vi "Periodic Tasks.vi"(8 "error in":errorcluster) -> ()   [LabVIEW 2016]
doc: "This VI runs in parallel to other tasks. It can contain as many user-defined periodic loops as you need. These can carry out PID or other sorts of timed response."
uses:
  <vilib>/Rock Robotics/WPI/Solenoid/WPI_SolenoidValue.ctl
  <vilib>/Rock Robotics/WPI/Utilities/WPI_GetSetVariantRefNum.vi
  Robot Global Data.vi
  <vilib>/addons/control/pid/pid.llb/PID (DBL).vi
  <vilib>/Rock Robotics/WPI/RobotDrive/WPI_RobotDriveMecanumDrive_Cartesian.vi
  <vilib>/Rock Robotics/WPI/Solenoid/WPI_SolenoidSetEnum.vi
  <vilib>/Rock Robotics/Network Tables/NT Read Number.vi
  <vilib>/Rock Robotics/Network Tables/NT Write Boolean.vi
  navX Library v2/navX Library v2.lvlib
  <vilib>/Analysis/NI_AALBase.lvlib
  <vilib>/addons/control/pid/NI_PID_pid.lvlib
panel:
  in  "gearDepthresh left":dbl=1.92 format="%#_13g"
  out "target angle":dbl
  in  "cam FOV":dbl=34.0 format="%#_13g"
  out "panic":bool
  out "YavSaved":dbl=162.56
  in  "PID Strafe Straight":T1={"proportional gain (Kc)"=0.05, "integral time (Ti, min)"=0.007, "derivative time (Td, min)"=0.001} {"derivative time (Td, min)" format="%.3f"; "integral time (Ti, min)" format="%.3f"; "proportional gain (Kc)" format="%.3f"}
  in  "min thresh 2":dbl=5e-05 format="%#_13g"
  in  "add if slow 2":dbl=0.005 format="%#_13g"
  in  "add if fast 2":dbl format="%#_13g"
  in  "min thresh":dbl=5e-05 format="%#_13g"
  in  "add if slow":dbl=0.005 format="%#_13g"
  in  "add if fast":dbl format="%#_13g"
  in  "aim thresh fast to mid":dbl=90.0
  out "turnSpeedSlow working":dbl=0.18
  out "turnSpeedStartSlow working":dbl=0.17
  in  "turnSpeedMedium":dbl=0.2 format="%#_13g"
  in  "turnSpeedHard":dbl=0.25 format="%#_13g"
  in  "cameraTarget":dbl=-0.195 format="%#_13g"
  in  "aim thresh start as slow":dbl=15.0 format="%#_13g"
  in  "turnSpeedSlow":dbl=0.19 format="%#_13g"
  in  "turnSpeedStartSlow":dbl=0.19
  out "aimState":i32
  out "leftOrRight":dbl=1.0
  in  "aim thresh mid to slow":dbl=30.0
  out "aimBot":dbl
  in  "hopperSpeedClose":dbl=0.5 step=0.05
  in  "Kd 2":dbl
  in  "Ki 2":dbl
  in  "Kp 2":dbl
  in  "armPanic Thresh":dbl=1.0
  in  "gearDepthresh right":dbl=1.92 format="%#_13g"
  out "std dev":dbl=3.505907882345
  out "mean":dbl=4.613466334164588
  in  "gearSensthresh":dbl=1.15 format="%#_13g"
  out "Input Voltage":dbl=10.350000000000001
  out "voltage (V)":dbl=10.15
  in  "SHIMMYTIME2":i32=10
  in  "SHIMMYTIME1":i32=10
  out "Waveform Graph":dbl[](graph)=[0.0, 0.0, 0.0, 0.0, 0.0, 0.0, 0.0, 0.0, 0.0, 0.0, 0.0, 0.0, 0.0, 0.0, 0.0, 0.0, 0.0, 0.0, 0.0, 0.0, 0.0, 0.0, 0.0, 0.0, 0.0, 0.0, 0.0, 0.0, 0.0, 0.0, 0.0, 0.0, 0.0, 0.0, 0.0, 0.0, 0.0, 0.0, 0.0, 0.0, 0.0, 0.0, 0.0, 0.0, 0.0, 0.0, 0.0, 0.0, 0.0, 0.0, 0.0, 0.0, 0.0, 0.0, 0.0, 0.0, 0.0, 0.0, 0.0, 0.0, 0.0, 0.0, 0.0, 0.0, 0.0, 0.0, 0.0, 0.0, 0.0, 0.0, 0.0, 0.0, 0.0, 0.0, 0.0, 0.0, 0.0, 0.0, 0.0, 0.0, 0.0, 0.0, 0.0, 0.0, 0.0, 0.0, 0.0, 0.0, 0.0, 0.0, 0.0, 0.0, 0.0, 0.0, 0.0, 0.0, 0.0, 0.0, 0.0, 0.0, 0.0, 0.0, 0.0, 0.0, 0.0, 0.0, 0.0, 0.0, 0.0, 0.0, 0.0, 0.0, 0.0, 0.0, 0.0, 0.0, 0.0, 0.0, 0.0, 0.0, 0.0, 0.0, 0.0, 0.0, 0.0, 0.0, 0.0, 0.0, 0.0, 0.0, 0.0, 0.0, 0.0, 0.0, 0.0, 0.0, 0.0, 0.0, 0.0, 0.0, 0.0, 0.0, 0.0, 0.0, 5.625, 5.875, 6.125, 6.0, 6.0, 6.0, 7.0, 8.0, 7.5, 7.0, 6.75, 6.5, 6.625, 6.25, 9.625, 10.25, 6.875, 6.625, 6.75, 7.125, 6.875, 6.875, 6.875, 7.0, 6.625, 7.125, 6.625, 6.375, 6.875, 7.5, 7.125, 7.875, 8.75, 8.25, 6.75, 7.375, 7.125, 7.375, 7.125, 7.125, 6.625, 6.5, 7.0, 7.0, 7.0, 6.75, 7.125, 7.625, 7.0, 7.75, 7.0, 7.125, 6.625, 7.25, 6.625, 6.75, 6.75, 6.75, 6.75, 7.0, 6.5, 6.75, 7.625, 7.25, 7.25, 7.25, 6.5, 7.0, 6.875, 7.125, 7.0, 7.25, 7.375, 6.875, 6.625, 6.625, 7.25, 6.5, 7.0, 6.75, 6.375, 6.75, 6.75, 6.875, 6.75, 6.75, 6.875, 6.25, 7.0, 6.375, 6.375, 6.875, 7.0, 6.5, 7.875, 8.5, 6.75, 6.625, 7.0, 7.0, 6.875, 7.0, 6.875, 8.125, 7.375, 6.75, 6.5, 6.375, 6.375, 6.875, 6.75, 7.0, 7.125, 7.125, 6.875, 7.0, 7.125, 7.875, 7.875, 8.75, 8.25, 7.0, 7.625, 7.0, 7.25, 7.125, 7.25, 7.0, 6.875, 7.0, 6.875, 7.25, 7.75, 7.625, 7.25, 7.125, 8.0, 8.75, 7.25, 7.125, 8.125, 10.125, 9.5, 8.75, 7.0, 6.875, 6.75, 6.875, 6.75, 7.25, 7.0, 8.25, 7.875, 7.5, 7.875, 6.75, 6.75, 7.875, 8.0, 8.375, 7.0, 6.75, 8.75, 7.875, 7.5, 7.5, 8.5, 7.0, 6.75, 7.125, 7.5, 7.375, 7.625, 7.25, 7.0, 6.875, 7.0, 7.125, 7.125, 8.25, 7.625, 7.125, 7.375, 7.125, 7.0, 7.875, 6.875, 7.0, 7.25, 7.25, 6.75, 6.875, 7.5, 6.5, 7.0, 6.875, 6.75, 6.875, 7.0, 6.875, 7.0, 7.25, 7.75, 7.875, 6.75, 6.875, 7.375, 7.125, 6.625, 7.625, 7.0, 7.25, 7.125, 7.125, 7.25, 7.25, 7.5, 6.875, 6.75, 7.0, 6.75, 6.125, 7.125, 6.75, 6.75, 6.875, 7.875, 7.125, 7.375, 7.0, 6.625, 6.75, 7.875, 9.25, 10.125, 7.625, 7.125, 6.625, 7.125, 8.625, 8.5, 7.375, 7.0, 7.0, 7.375, 11.5, 6.875, 7.125, 6.875, 6.875, 7.5, 7.5, 7.625, 7.375, 6.875, 7.125, 7.25]
  in  "Kd":dbl
  in  "Ki":dbl
  in  "Kp":dbl
  in  "ARM Retainer open":bool
  in  "SEQ Retainer Open":bool
  in  "Gear Shover":bool
  in  "Ramp-Up":dbl format="%#_13g"
  out "Shooter Speed":dbl
  out "trim close":dbl=1.0009448818897637
  out "trim far":dbl=1.0003149606299213
  out "timeSaved 2":i32=400
  in  "drop gear time":i32=40
  in  "open retainer time":i32=20
  in  "shooter target speed close":dbl=6.5 format="%.2f"
  in  "feed forward close":dbl=0.66 step=0.05
  in  "shooter target speed far":dbl=7.0 format="%.2f"
  out "timeSaved":i32=41241
  in  "shimmyspeed":dbl=0.3
  in  "xshimmy":bool
  in  "intakeSpeed":dbl=0.8
  in  "Slews":cluster{"slewX":dbl, "slewYgo":dbl, "slewZ":dbl}={"slewX"=0.2, "slewYgo"=0.2, "slewZ"=0.15}
  # "DRIVE STUFF"
  # "BALL STUFF"
  # "GEAR STUFF"
  # ".5"
  # "2/16:\nFF far:      0.71\nFF Close: 0.66\nKp Far = 0.025\nTarget speed far = 7"
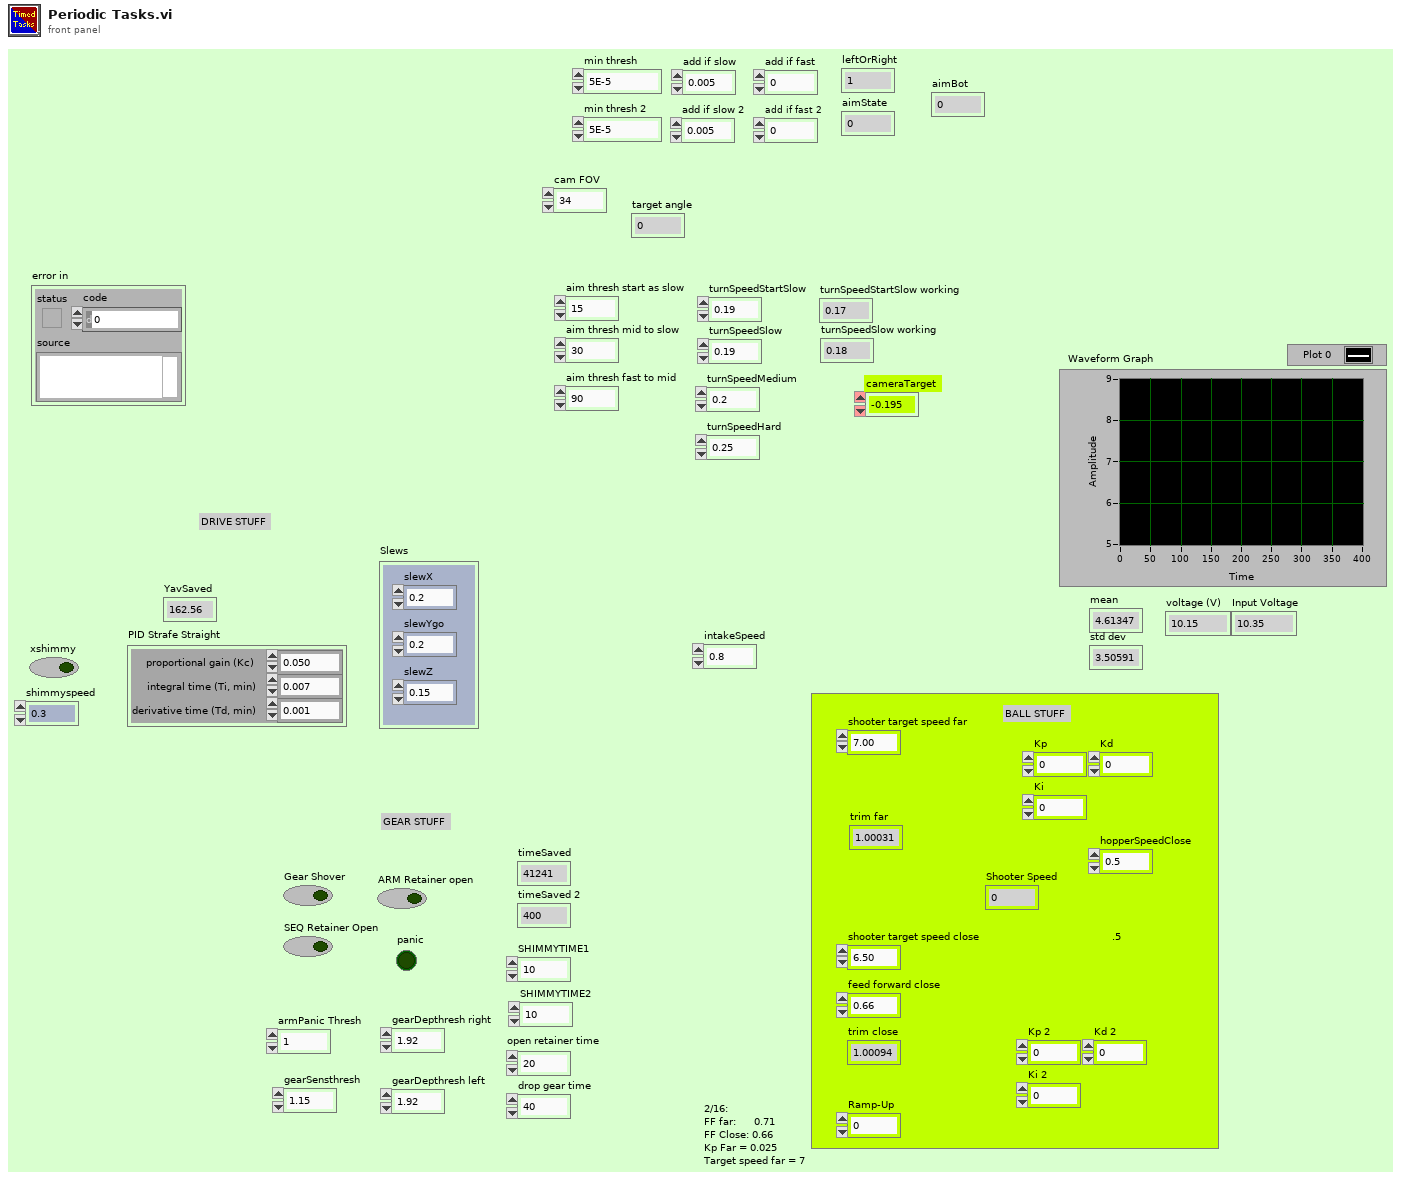
[diagram p1: front panel]
types:
  T1 = cluster{"proportional gain (Kc)":dbl, "integral time (Ti, min)":dbl, "derivative time (Td, min)":dbl}
  T2 = typedef "WPI_SolenoidDevRef.ctl" = cluster{"DevStatus":errorcluster, "Pneumatics Control Module":u8, "Forward Solenoid Channel":T3, "Reverse Solenoid Channel":T3}
  T3 = typedef "WPI_SolenoidChannel.ctl" = enum8{"Solenoid 0", "Solenoid 1", "Solenoid 2", "Solenoid 3", "Solenoid 4", "Solenoid 5", "Solenoid 6", "Solenoid 7", "Invalid"}
  T4 = typedef "navX Library v2.lvlib/Z900_navX_DeviceTypeDef.ctl" = cluster{"Interface":cluster{"Protocol":T5, "Update Rate (4Hz-100Hz)":u8, "navX Open TypeDef":variant}, "Notify Packet":refnum<notifier>, "Loop VI Refnum":refnum<vi>, "Ready to Close Occurrence Refnum":refnum<k4>}
  T5 = typedef "navX Library v2.lvlib/Z900_navX_ProtocolTypeDef.ctl" = enum16{"SERIAL", "I2C", "SPI"}
  T6 = typedef "WPI_EncoderDevRef.ctl" = cluster{"DevStatus":errorcluster, "EncoderIndex":T7, "CounterIndex":T8, "DistancePerCount":dbl, "Decoding Type":T9}
  T7 = typedef "FPGA_EncoderIdx.ctl" = enum8{"Enc 0", "Enc 1", "Enc 2", "Enc 3", "Enc 4", "Enc 5", "Enc 6", "Enc 7", "Invalid"}
  T8 = typedef "FPGA_CounterCtrSystemIndex.ctl" = enum8{"Ctr 0", "Ctr 1", "Ctr 2", "Ctr 3", "Ctr 4", "Ctr 5", "Ctr 6", "Ctr 7", "Invalid"}
  T9 = typedef "WPI_EncoderType.ctl" = enum16{"1x", "2x", "4x"}
  T10 = typedef "WPI_MotorControlDeviceRef.ctl" = cluster{"DeviceStatus":errorcluster, "Type":T11, "PWM":cluster{"PWM Channel":T12, "DeadBand":T13}, "CAN":cluster{"Device Number":u8, "SetOutput VI Ref":variant, "GetOutput VI Ref":variant, "Enable VI Ref":variant, "Disable VI Ref":variant, "Data":variant}, "Invert":bool}
  T11 = typedef "WPI_MotorControlType.ctl" = enum16{"PWM", "CAN"}
  T12 = typedef "FPGA_DIOPWMChannel.ctl" = enum8{"PWM 0", "PWM 1", "PWM 2", "PWM 3", "PWM 4", "PWM 5", "PWM 6", "PWM 7", "PWM 8", "PWM 9", "PWM MXP 0", "PWM MXP 1", "PWM MXP 2", "PWM MXP 3", "PWM MXP 4", "PWM MXP 5", "PWM MXP 6", "PWM MXP 7", "PWM MXP 8", "PWM MXP 9", "Invalid"}
  T13 = typedef "WPI_PWMDeadband.ctl" = cluster{"Name":string, "maxPositivePwm":i32, "minPositivePwm":i32, "centerPwm":i32, "maxNegativePwm":i32, "minNegativePwm":i32, "angularRange":u16}
  T14 = typedef "WPI_CompressorDevRef.ctl" = cluster{"DevStatus":errorcluster, "Pneumatics Control Module":u8}
  T15 = typedef "WPI_RobotDriveDevRef.ctl" = cluster{"DevStatus":errorcluster, "Motors[]":T10[], "Square Inputs":bool, "Max Output":dbl}
  T16 = typedef "WPI_AnalogChannelDevRef.ctl" = cluster{"DevStatus":errorcluster, "Analog Channel":T17}
  T17 = typedef "FPGA_AIChannel.ctl" = enum8{"AI 0", "AI 1", "AI 2", "AI 3", "AI MXP 0", "AI MXP 1", "AI MXP 2", "AI MXP 3", "Invalid"}
  T18 = cluster{"Yaw":dbl, "Roll":dbl, "Pitch":dbl, "Heading":dbl, "Fused Heading":dbl}
  T19 = typedef "WPI_SolenoidValue.ctl" = enum16{"Off", "On", "Forward", "Reverse"}
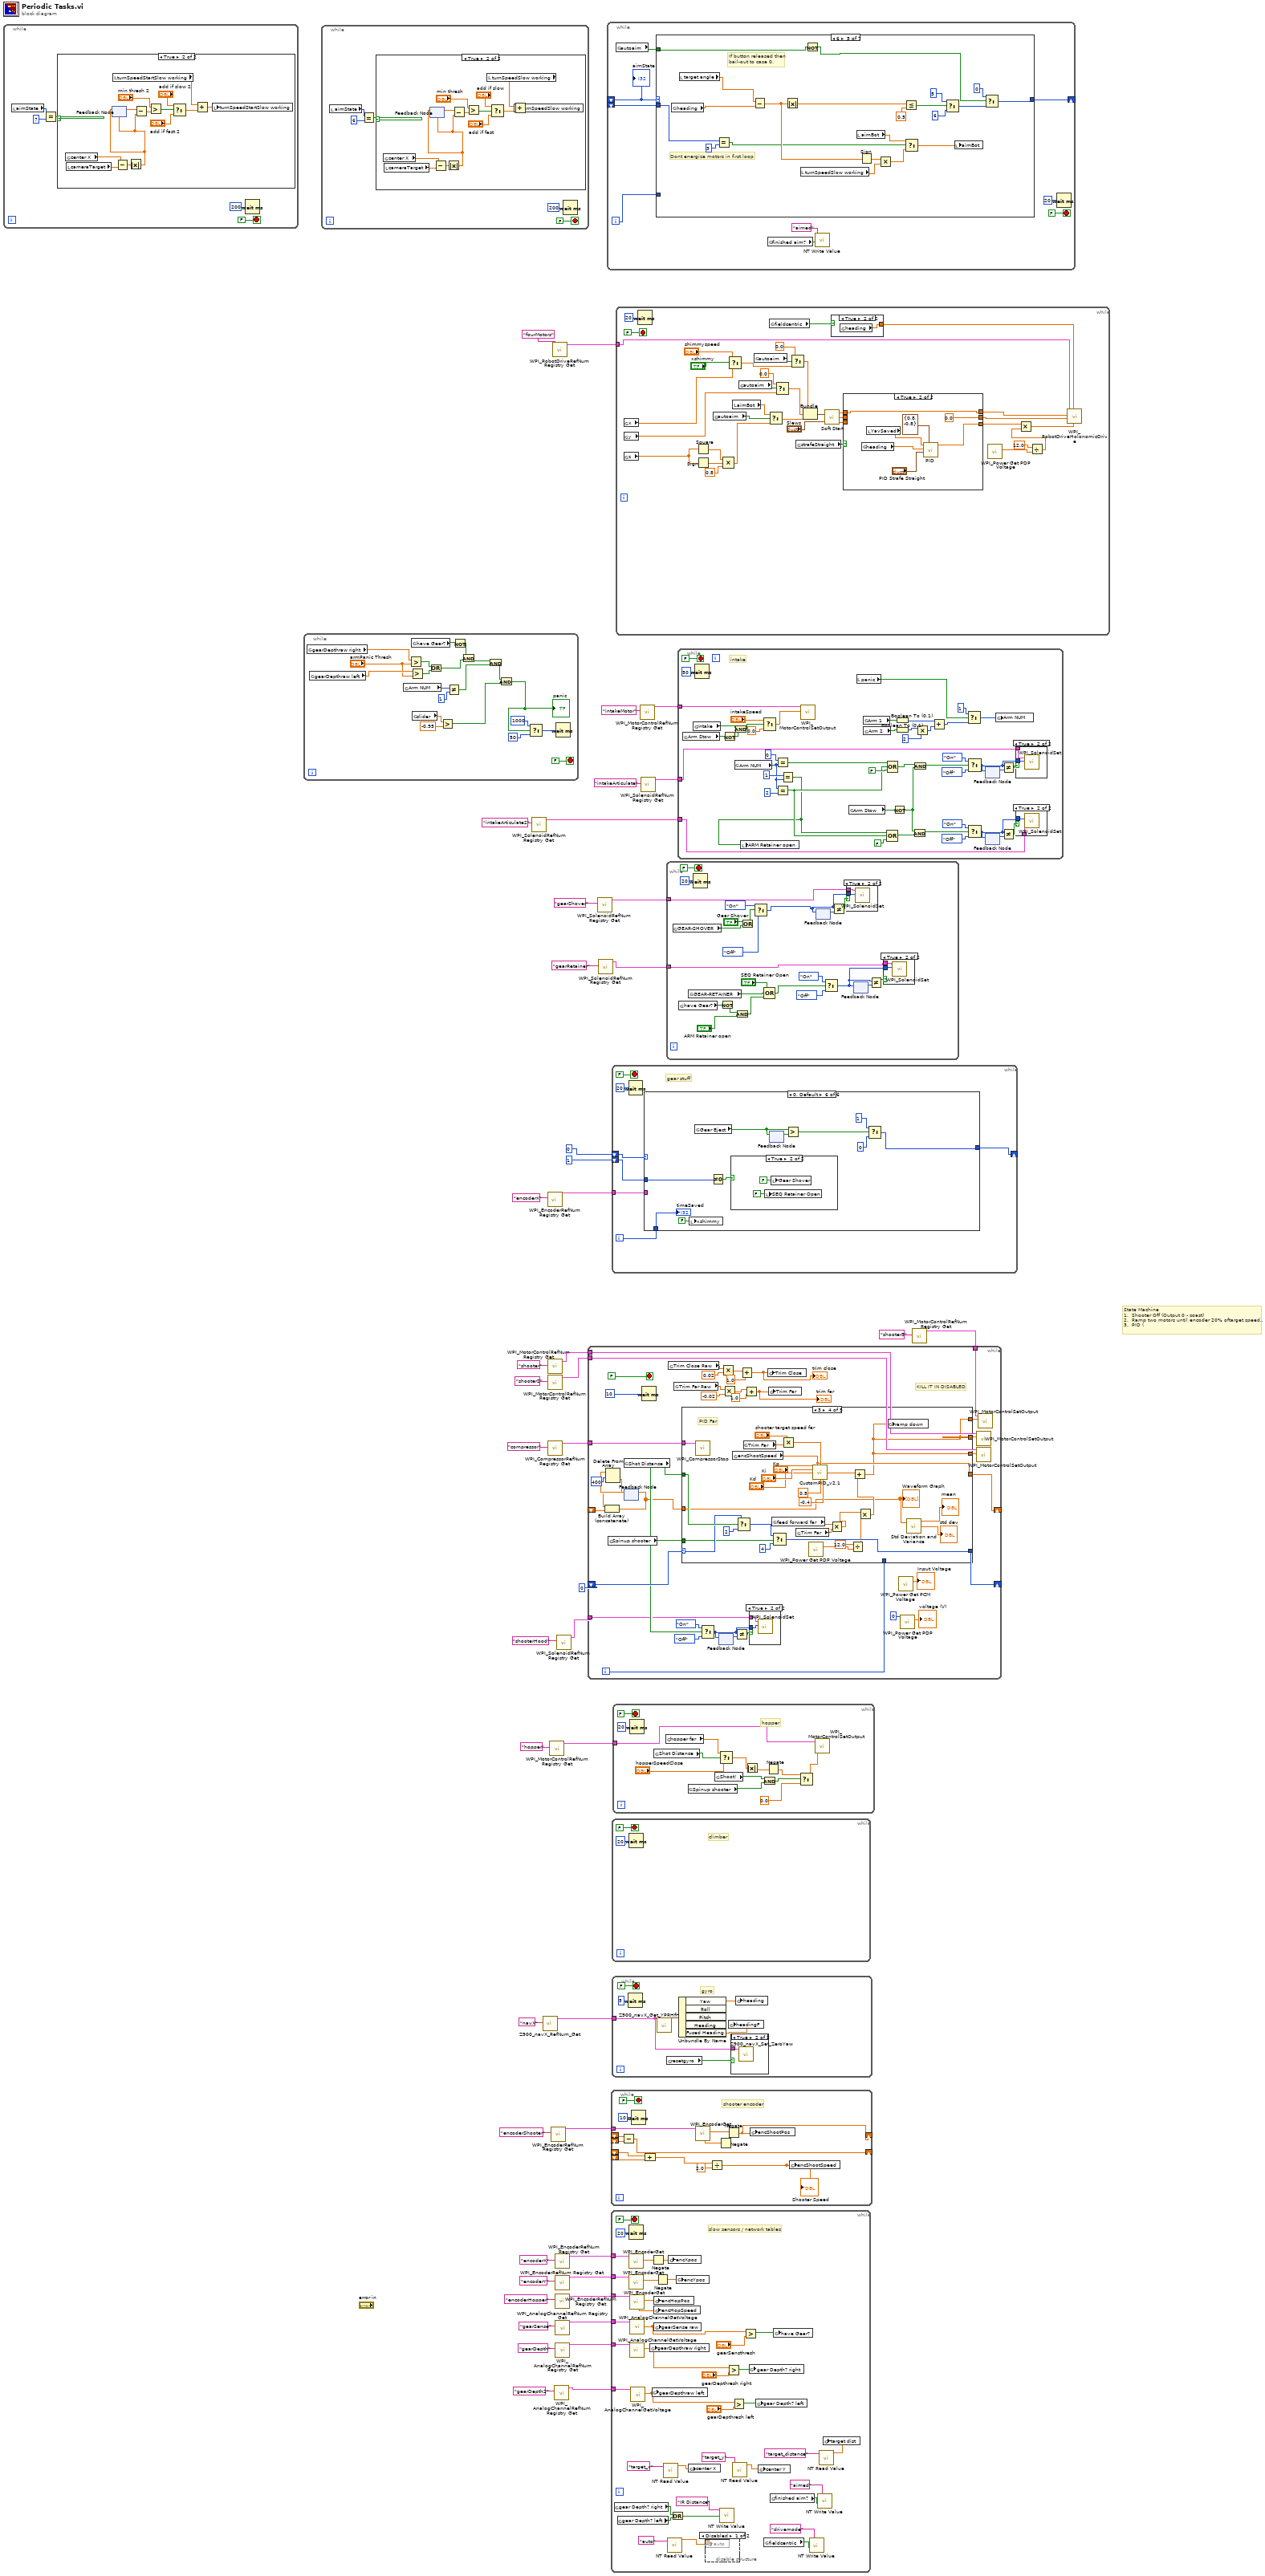
[diagram p0: block diagram]
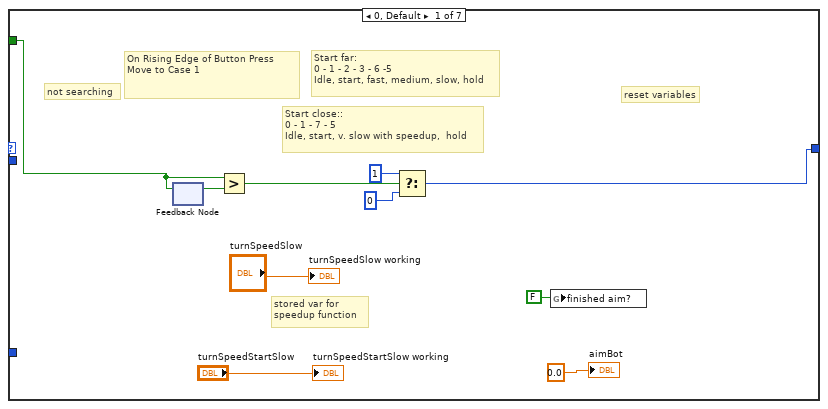
[diagram p4: hidden frame]
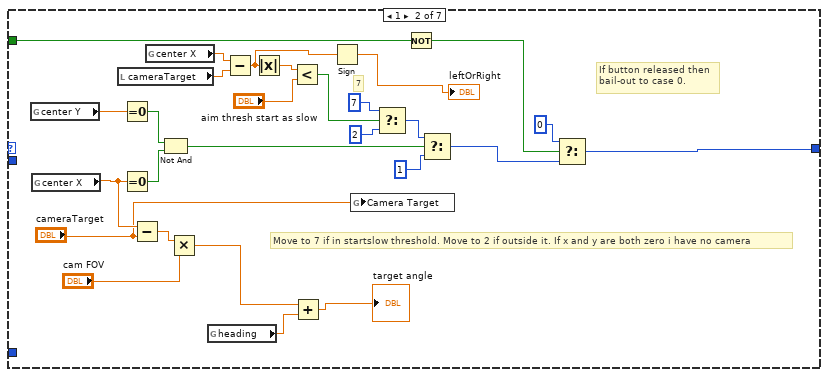
[diagram p5: hidden frame]
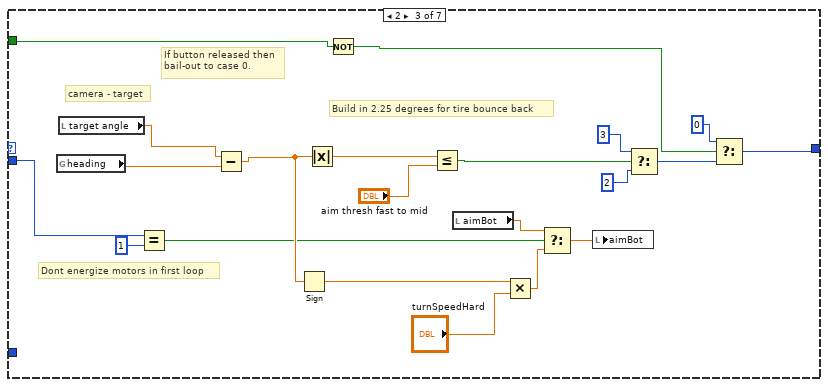
[diagram p6: hidden frame]
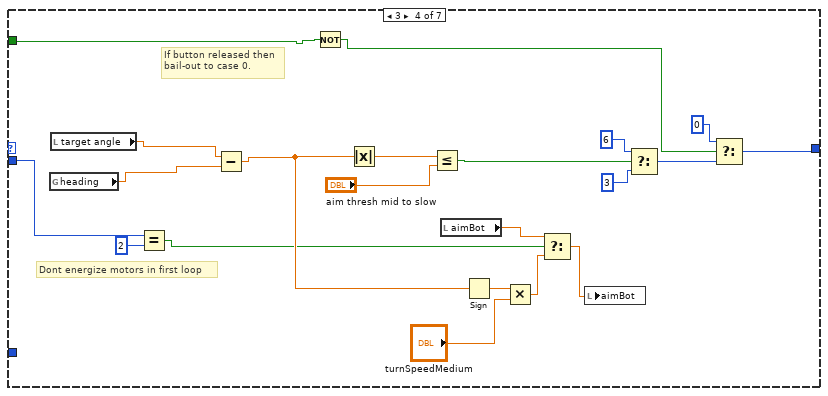
[diagram p7: hidden frame]
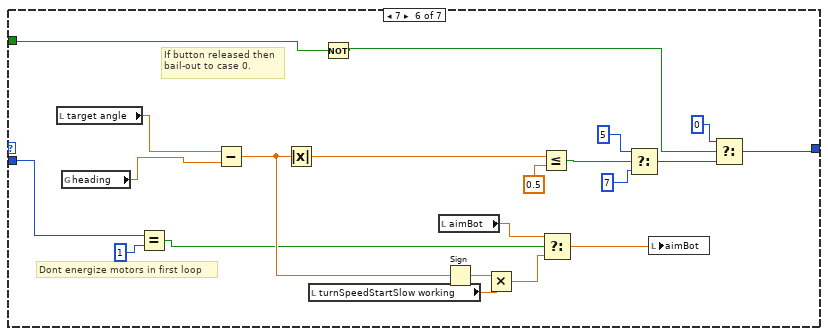
[diagram p8: hidden frame]
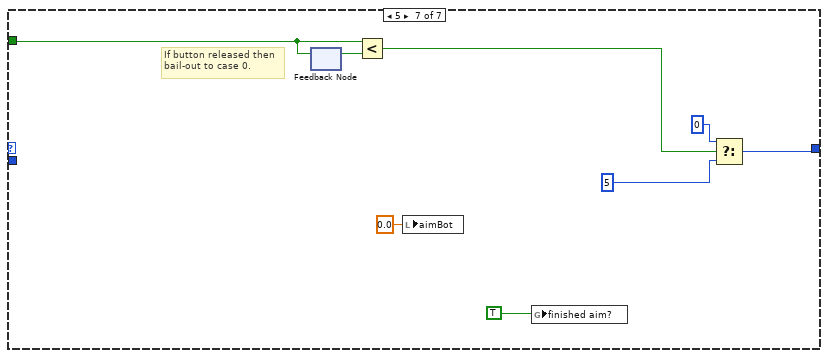
[diagram p9: hidden frame]
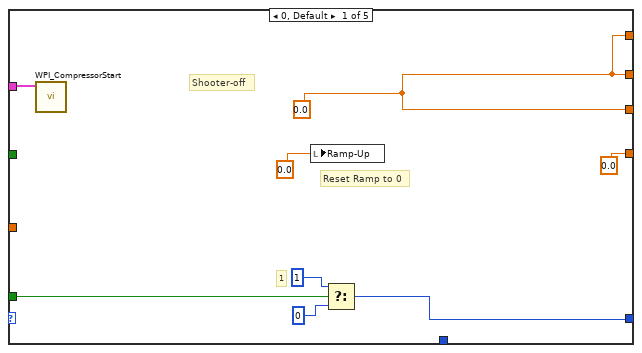
[diagram p15: hidden frame]
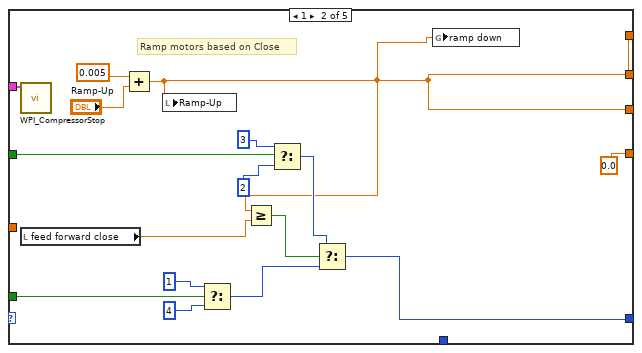
[diagram p16: hidden frame]
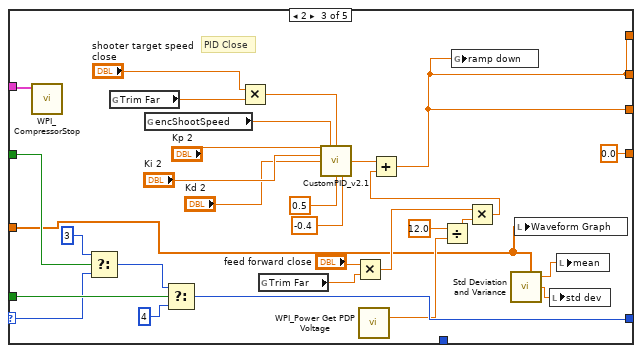
[diagram p17: hidden frame]
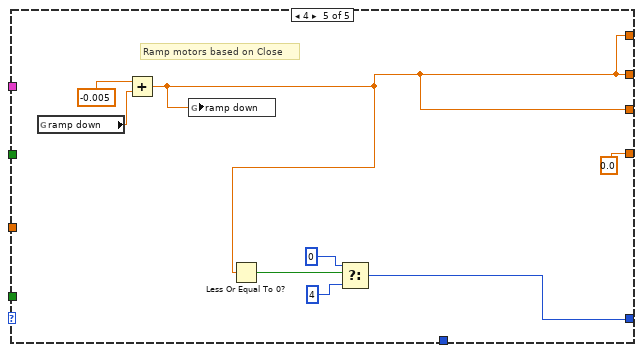
[diagram p18: hidden frame]
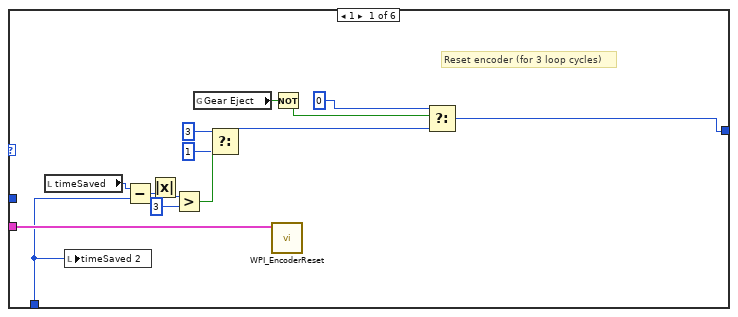
[diagram p19: hidden frame]
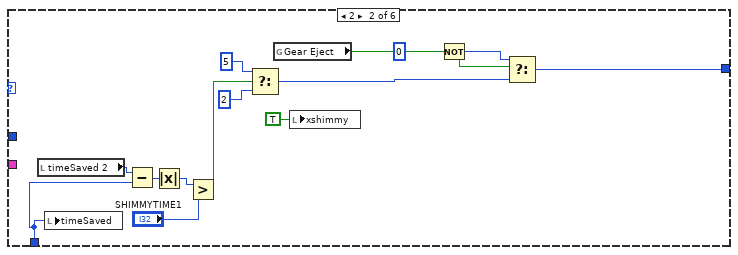
[diagram p20: hidden frame]
diagram:
  # "State Machine\n1.  Shooter Off (Output 0 - coast)\n2.  Ramp two motors until encoder 20% oftarget speed..\n3.  PID ("
  n1 = while {
    stop <- FALSE stop-if-true
    n2 = local read "aimState"() -> (w48:i32)
    n3 = Equal?(x=w48, y=7) -> (x = y?=w46:bool)
    n4 = case shown="True" w46 {
      frame False {
      }
      frame True {
        n5 = global read "Robot Global Data.vi" "center X"() -> (w63:dbl)
        n6 = local read "cameraTarget"() -> (w62:dbl)
        n7 = local read "turnSpeedStartSlow working"() -> (w54:dbl)
        n8 = Subtract(x=w63, y=w62) -> (x-y=w52:dbl)
        n9 = Absolute Value(x=w52) -> (abs(x)=w51:dbl)
        n10 = feedback #1(w51) -> (w60:dbl)
        n11 = feedback-in #1(w51) -> ()
        n12 = Subtract(x=w60, y=w51) -> (x-y=w59:dbl)
        n13 = Greater?(x="min thresh 2", y=w59) -> (0:w57:bool)
        n14 = Select(t="add if slow 2", s=w57, f="add if fast 2") -> (s? t:f=w55:dbl)
        n15 = Add(x=w54, y=w55) -> (x+y=w53:dbl)
        n16 = local write "turnSpeedStartSlow working"(w53) -> ()
      }
    }
    n17 = Wait (ms)(milliseconds to wait=u32 200) -> ()  [unwired: 1 out]
  }
  n18 = while {
    stop <- FALSE stop-if-true
    n19 = global read "Robot Global Data.vi" "gearDepthraw right"() -> (w83:dbl)
    n20 = global read "Robot Global Data.vi" "gearDepthraw left"() -> (w69:dbl)
    n21 = global read "Robot Global Data.vi" "Arm NUM"() -> (w76:i16)
    n22 = Greater?(x=w83, y="armPanic Thresh") -> (0:w66:bool)
    n23 = Greater?(x=w69, y="armPanic Thresh") -> (0:w65:bool)
    n24 = global read "Robot Global Data.vi" "have Gear?"() -> (w82:bool)
    n25 = global read "Robot Global Data.vi" "slider"() -> (w73:dbl)
    n26 = Or(x=w66, y=w65) -> (x .or. y?=w64:bool)
    n27 = Greater?(x=w73, y=-0.95) -> (0:w71:bool)
    n28 = Not Equal?(x=w76, y=i16 1) -> (x != y?=w77:bool)
    n29 = Not(x=w82) -> (.not. x?=w67:bool)
    n30 = And(x=w67, y=w64) -> (x .and. y?=w78:bool)
    n31 = And(x=w78, y=w77) -> (x .and. y?=w74:bool)
    n32 = And(x=w74, y=w71) -> (x .and. y?=w70:bool)
    "panic" <- w70
    n33 = Select(t=u32 1000, s=w70, f=u32 50 ("milliseconds to wait")) -> (s? t:f=w81:u32)
    n34 = Wait (ms)(milliseconds to wait=w81) -> ()  [unwired: 1 out]
  }
  n35 = while {
    stop <- FALSE stop-if-true
    n36 = local read "aimState"() -> (w87:i32)
    n37 = Equal?(x=w87, y=6) -> (x = y?=w85:bool)
    n38 = case shown="True" w85 {
      frame False {
      }
      frame True {
        n39 = global read "Robot Global Data.vi" "center X"() -> (w102:dbl)
        n40 = local read "cameraTarget"() -> (w101:dbl)
        n41 = Subtract(x=w102, y=w101) -> (x-y=w91:dbl)
        n42 = Absolute Value(x=w91) -> (abs(x)=w90:dbl)
        n43 = feedback #2(w90) -> (w99:dbl)
        n44 = feedback-in #2(w90) -> ()
        n45 = Subtract(x=w99, y=w90) -> (x-y=w98:dbl)
        n46 = Greater?(x="min thresh", y=w98) -> (0:w96:bool)
        n47 = local read "turnSpeedSlow working"() -> (w93:dbl)
        n48 = Select(t="add if slow", s=w96, f="add if fast") -> (s? t:f=w94:dbl)
        n49 = Add(x=w93, y=w94) -> (x+y=w92:dbl)
        n50 = local write "turnSpeedSlow working"(w92) -> ()
      }
    }
    n51 = Wait (ms)(milliseconds to wait=u32 200) -> ()  [unwired: 1 out]
  }
  n52 = call <vilib>:"WPI_SolenoidRefNum Registry Get.vi"("refnum name"="intakeArticulate2") -> ("SolenoidDevRef"=w38:T2)  [unwired: 9 in, 1 out]
  n53 = call "Z900_navX_RefNum_Get.vi"("refnum name"="navX") -> ("navX Device"=w18:T4)  [unwired: 9 in, 1 out]
  n54 = call <vilib>:"WPI_EncoderRefNum Registry Get.vi"("refnum name"="encoderX") -> ("EncoderDevRef"=w35:T6)  [unwired: 9 in, 1 out]
  n55 = call <vilib>:"WPI_MotorControlRefNum Registry Get.vi"("refnum name"="shooter") -> ("MotorControlDevRef"=w28:T10)  [unwired: 9 in, 1 out]
  n56 = call <vilib>:"WPI_MotorControlRefNum Registry Get.vi"("refnum name"="shooter2") -> ("MotorControlDevRef"=w27:T10)  [unwired: 9 in, 1 out]
  n57 = call <vilib>:"WPI_CompressorRefNum Registry Get.vi"("refnum name"="compressor") -> ("CompressorDevRef"=w24:T14)  [unwired: 9 in, 1 out]
  n58 = call <vilib>:"WPI_MotorControlRefNum Registry Get.vi"("refnum name"="hopper") -> ("MotorControlDevRef"=w25:T10)  [unwired: 9 in, 1 out]
  n59 = call <vilib>:"WPI_EncoderRefNum Registry Get.vi"("refnum name"="encoderShooter") -> ("EncoderDevRef"=w9:T6)  [unwired: 9 in, 1 out]
  n60 = call <vilib>:"WPI_RobotDriveRefNum Registry Get.vi"("refnum name"="fourMotors") -> ("RobotDriveDevRef"=w44:T15)  [unwired: 1 in, 9 out]
  n61 = call <vilib>:"WPI_AnalogChannelRefNum Registry Get.vi"("refnum name"="gearDepth2") -> ("AIDeviceRef"=w1:T16)  [unwired: 9 in, 1 out]
  n62 = call <vilib>:"WPI_EncoderRefNum Registry Get.vi"("refnum name"="encoderX") -> ("EncoderDevRef"=w15:T6)  [unwired: 9 in, 1 out]
  n63 = call <vilib>:"WPI_EncoderRefNum Registry Get.vi"("refnum name"="encoderY") -> ("EncoderDevRef"=w11:T6)  [unwired: 9 in, 1 out]
  n64 = call <vilib>:"WPI_EncoderRefNum Registry Get.vi"("refnum name"="encoderHopper") -> ("EncoderDevRef"=w10:T6)  [unwired: 9 in, 1 out]
  n65 = call <vilib>:"WPI_AnalogChannelRefNum Registry Get.vi"("refnum name"="gearSense") -> ("AIDeviceRef"=w6:T16)  [unwired: 9 in, 1 out]
  n66 = call <vilib>:"WPI_AnalogChannelRefNum Registry Get.vi"("refnum name"="gearDepth") -> ("AIDeviceRef"=w5:T16)  [unwired: 9 in, 1 out]
  n67 = call <vilib>:"WPI_SolenoidRefNum Registry Get.vi"("refnum name"="shooterHood") -> ("SolenoidDevRef"=w29:T2)  [unwired: 9 in, 1 out]
  n68 = call <vilib>:"WPI_SolenoidRefNum Registry Get.vi"("refnum name"="gearShover") -> ("SolenoidDevRef"=w20:T2)  [unwired: 9 in, 1 out]
  n69 = call <vilib>:"WPI_SolenoidRefNum Registry Get.vi"("refnum name"="gearRetainer") -> ("SolenoidDevRef"=w19:T2)  [unwired: 9 in, 1 out]
  n70 = while {
    shift-right: [w110] -> _
    shift-left: _ -> [w108]
    shift-left: _ -> [w105]
    i -> [w106]
    stop <- FALSE stop-if-true
    n71 = global read "Robot Global Data.vi" "autoaim"() -> (w109:bool)
    n72 = case shown="6" w108 {
      tunnel: w109 -> [w115 w130 w151 w172 w194 w215 w237]
      tunnel: [w119 w147 w165 w187 w207 w228 w236] -> w110
      tunnel: w106 -> [_ _ _ _ _ _ _]
      tunnel: w105 -> [_ _ w158 w182 w193 w224 _]
      frame 0, Default {
        # "Start close::\n0 - 1 - 7 - 5\nIdle, start, v. slow with speedup,  hold"
        # "Start far:\n0 - 1 - 2 - 3 - 6 -5\nIdle, start, fast, medium, slow, hold"
        # "stored var for\nspeedup function"
        # "On Rising Edge of Button Press\nMove to Case 1"
        # "reset variables"
        # "not searching"
        n73 = feedback #3() -> (w121:bool)  [unwired: 1 in]
        n74 = feedback-in #3(w115) -> ()
        n75 = Greater?(x=w115, y=w121) -> (0:w118:bool)
        n76 = Select(t=1, s=w118, f=0) -> (s? t:f=w119:i32)
        n77 = global write "Robot Global Data.vi" "finished aim?"(FALSE ("4?")) -> ()
        "aimBot" <- 0.0 ("aimBot")
        "turnSpeedSlow working" <- "turnSpeedSlow"
        "turnSpeedStartSlow working" <- "turnSpeedStartSlow"
      }
      frame 1 {
        # "7"
        # "Move to 7 if in startslow threshold. Move to 2 if outside it. If x and y are both zero i have no camera"
        # "If button released then\nbail-out to case 0."
        n78 = global read "Robot Global Data.vi" "center Y"() -> (w145:dbl)
        n79 = global read "Robot Global Data.vi" "center X"() -> (w128:dbl)
        n80 = local read "cameraTarget"() -> (w139:dbl)
        n81 = Equal To 0?(x=w145) -> (x = 0?=w143:bool)
        n82 = Equal To 0?(x=w128) -> (x = 0?=w144:bool)
        n83 = Subtract(x=w128, y="cameraTarget") -> (x-y=w127:dbl)
        n84 = global read "Robot Global Data.vi" "center X"() -> (w138:dbl)
        n85 = Not And(1:w144, 2:w143) -> (0:w142:bool)
        n86 = Multiply(x=w127, y="cam FOV") -> (x*y=w123:dbl)
        n87 = global read "Robot Global Data.vi" "heading"() -> (w122:dbl)
        n88 = Subtract(x=w138, y=w139) -> (x-y=w132:dbl)
        n89 = Absolute Value(x=w132) -> (abs(x)=w137:dbl)
        n90 = Less?(x=w137, y="aim thresh start as slow") -> (x < y?=w135:bool)
        n91 = Add(x=w123, y=w122) -> (x+y=→"target angle":dbl)
        n92 = Sign(1:w132) -> (0:→"leftOrRight":dbl)
        n93 = global write "Robot Global Data.vi" "Camera Target"("cameraTarget") -> ()
        n94 = Select(t=7, s=w135, f=2) -> (s? t:f=w133:i32)
        n95 = Not(x=w130) -> (.not. x?=w129:bool)
        n96 = Select(t=w133, s=w142, f=1) -> (s? t:f=w141:i32)
        n97 = Select(t=0, s=w129, f=w141) -> (s? t:f=w147:i32)
      }
      frame 2 {
        # "camera - target"
        # "Build in 2.25 degrees for tire bounce back"
        # "Dont energize motors in first loop"
        # "If button released then\nbail-out to case 0."
        n98 = global read "Robot Global Data.vi" "heading"() -> (w150:dbl)
        n99 = local read "target angle"() -> (w149:dbl)
        n100 = Equal?(x=w158, y=1) -> (x = y?=w156:bool)
        n101 = Subtract(x=w149, y=w150) -> (x-y=w161:dbl)
        n102 = Sign(1:w161) -> (0:w162:dbl)
        n103 = Absolute Value(x=w161) -> (abs(x)=w163:dbl)
        n104 = Not(x=w151) -> (.not. x?=w152:bool)
        n105 = Less Or Equal?(x=w163, y="aim thresh fast to mid") -> (x <= y?=w164:bool)
        n106 = local read "aimBot"() -> (w155:dbl)
        n107 = Multiply(x=w162, y="turnSpeedHard") -> (x*y=w160:dbl)
        n108 = Select(t=w155, s=w156, f=w160) -> (s? t:f=w159:dbl)
        n109 = local write "aimBot"(w159) -> ()
        n110 = Select(t=3, s=w164, f=2) -> (s? t:f=w167:i32)
        n111 = Select(t=0, s=w152, f=w167) -> (s? t:f=w165:i32)
      }
      frame 3 {
        # "Dont energize motors in first loop"
        # "If button released then\nbail-out to case 0."
        n112 = global read "Robot Global Data.vi" "heading"() -> (w171:dbl)
        n113 = local read "target angle"() -> (w170:dbl)
        n114 = Equal?(x=w182, y=2) -> (x = y?=w180:bool)
        n115 = Subtract(x=w170, y=w171) -> (x-y=w185:dbl)
        n116 = Not(x=w172) -> (.not. x?=w173:bool)
        n117 = Absolute Value(x=w185) -> (abs(x)=w186:dbl)
        n118 = Less Or Equal?(x=w186, y="aim thresh mid to slow") -> (x <= y?=w175:bool)
        n119 = local read "aimBot"() -> (w179:dbl)
        n120 = Sign(1:w185) -> (0:w177:dbl)
        n121 = Multiply(x=w177, y="turnSpeedMedium") -> (x*y=w184:dbl)
        n122 = Select(t=w179, s=w180, f=w184) -> (s? t:f=w183:dbl)
        n123 = local write "aimBot"(w183) -> ()
        n124 = Select(t=6, s=w175, f=3) -> (s? t:f=w189:i32)
        n125 = Select(t=0, s=w173, f=w189) -> (s? t:f=w187:i32)
      }
      frame 6 {
        # "Dont energize motors in first loop"
        # "If button released then\nbail-out to case 0."
        n126 = global read "Robot Global Data.vi" "heading"() -> (w192:dbl)
        n127 = local read "target angle"() -> (w191:dbl)
        n128 = Equal?(x=w193, y=3) -> (x = y?=w201:bool)
        n129 = Subtract(x=w191, y=w192) -> (x-y=w204:dbl)
        n130 = Absolute Value(x=w204) -> (abs(x)=w196:dbl)
        n131 = local read "turnSpeedSlow working"() -> (w197:dbl)
        n132 = Not(x=w194) -> (.not. x?=w195:bool)
        n133 = local read "aimBot"() -> (w200:dbl)
        n134 = Sign(1:w204) -> (0:w205:dbl)
        n135 = Multiply(x=w205, y=w197) -> (x*y=w203:dbl)
        n136 = Less Or Equal?(x=w196, y=0.5 ("aimTolerance 2")) -> (x <= y?=w206:bool)
        n137 = Select(t=w200, s=w201, f=w203) -> (s? t:f=w198:dbl)
        n138 = Select(t=5, s=w206, f=6) -> (s? t:f=w209:i32)
        n139 = local write "aimBot"(w198) -> ()
        n140 = Select(t=0, s=w195, f=w209) -> (s? t:f=w207:i32)
      }
      frame 7 {
        # "Dont energize motors in first loop"
        # "If button released then\nbail-out to case 0."
        n141 = local read "target angle"() -> (w212:dbl)
        n142 = global read "Robot Global Data.vi" "heading"() -> (w213:dbl)
        n143 = Equal?(x=w224, y=1) -> (x = y?=w222:bool)
        n144 = Subtract(x=w212, y=w213) -> (x-y=w226:dbl)
        n145 = Absolute Value(x=w226) -> (abs(x)=w218:dbl)
        n146 = local read "turnSpeedStartSlow working"() -> (w214:dbl)
        n147 = Not(x=w215) -> (.not. x?=w216:bool)
        n148 = local read "aimBot"() -> (w221:dbl)
        n149 = Sign(1:w226) -> (0:w217:dbl)
        n150 = Multiply(x=w217, y=w214) -> (x*y=w225:dbl)
        n151 = Less Or Equal?(x=w218, y=0.5 ("aimTolerance 2")) -> (x <= y?=w227:bool)
        n152 = Select(t=w221, s=w222, f=w225) -> (s? t:f=w219:dbl)
        n153 = Select(t=5, s=w227, f=7) -> (s? t:f=w230:i32)
        n154 = local write "aimBot"(w219) -> ()
        n155 = Select(t=0, s=w216, f=w230) -> (s? t:f=w228:i32)
      }
      frame 5 {
        # "If button released then\nbail-out to case 0."
        n156 = feedback #4() -> (w239:bool)  [unwired: 1 in]
        n157 = feedback-in #4(w237) -> ()
        n158 = Less?(x=w237, y=w239) -> (x < y?=w238:bool)
        n159 = local write "aimBot"(0.0 ("aimBot")) -> ()
        n160 = global write "Robot Global Data.vi" "finished aim?"(TRUE ("4?")) -> ()
        n161 = Select(t=0, s=w238, f=5) -> (s? t:f=w236:i32)
      }
    }
    n162 = global read "Robot Global Data.vi" "finished aim?"() -> (w104:bool)
    n163 = call-poly <vilib>:"NT Write Value.vi"("Boolean"=w104, "Name"="aimed") -> ()  [unwired: 9 in, 1 out]
    n164 = Wait (ms)(milliseconds to wait=u32 20) -> ()  [unwired: 1 out]
    "aimState" <- w108
  }
  n165 = while {
    tunnel: w9 -> [w252]
    shift-right: [w246] -> _
    shift-left: _ -> [w245]
    shift-left: _ -> [w244]
    shift-right: [w243] -> _
    shift-left: _ -> [w242]
    shift-left: _ -> [w241]
    stop <- FALSE stop-if-true
    # "shooter encoder"
    n166 = Subtract(x=w245, y=w244) -> (x-y=w243:dbl)
    n167 = Wait (ms)(milliseconds to wait=u32 10) -> ()  [unwired: 1 out]
    n168 = Compound Arithmetic op=ADD(w242, w241) -> (w249:dbl)
    n169 = call <vilib>:"WPI_EncoderGet.vi"("EncoderDevRef"=w252) -> ("Distance"=w250:dbl, "Rate"=w251:dbl)  [unwired: 5 in, 4 out]
    n170 = Divide(x=w249, y=2.0) -> (x/y=w247:dbl)
    "Shooter Speed" <- w247
    n171 = Negate(x=w251) -> ()  [unwired: 1 out]
    n172 = Negate(x=w250) -> (-x=w246:dbl)
    n173 = global write "Robot Global Data.vi" "encShootPos"(w246) -> ()
    n174 = global write "Robot Global Data.vi" "encShootSpeed"(w247) -> ()
  }
  n175 = while {
    tunnel: w15 -> [w291]
    tunnel: w11 -> [w289]
    tunnel: w10 -> [w288]
    tunnel: w6 -> [w286]
    tunnel: w5 -> [w285]
    tunnel: w1 -> [w261]
    stop <- FALSE stop-if-true
    # "slow sensors / network tables"
    n176 = global read "Robot Global Data.vi" "gear Depth? right"() -> (w256:bool)
    n177 = global read "Robot Global Data.vi" "gear Depth? left"() -> (w257:bool)
    n178 = Wait (ms)(milliseconds to wait=u32 20) -> ()  [unwired: 1 out]
    n179 = call <vilib>:"WPI_EncoderGet.vi"("EncoderDevRef"=w291) -> ("Distance"=w272:dbl)  [unwired: 5 in, 5 out]
    n180 = call <vilib>:"WPI_EncoderGet.vi"("EncoderDevRef"=w289) -> ("Distance"=w270:dbl)  [unwired: 5 in, 5 out]
    n181 = call <vilib>:"WPI_EncoderGet.vi"("EncoderDevRef"=w288) -> ("Distance"=w290:dbl, "Rate"=w287:dbl)  [unwired: 5 in, 4 out]
    n182 = call <vilib>:"WPI_AnalogChannelGetVoltage.vi"("AIDeviceRef"=w285) -> ("Voltage"=w279:dbl)  [unwired: 8 in, 2 out]
    n183 = call <vilib>:"WPI_AnalogChannelGetVoltage.vi"("AIDeviceRef"=w286) -> ("Voltage"=w284:dbl)  [unwired: 8 in, 2 out]
    n184 = call <vilib>:"WPI_AnalogChannelGetVoltage.vi"("AIDeviceRef"=w261) -> ("Voltage"=w258:dbl)  [unwired: 8 in, 2 out]
    n185 = global write "Robot Global Data.vi" "gearDepthraw right"(w279) -> ()
    n186 = Negate(x=w272) -> (-x=w271:dbl)
    n187 = global write "Robot Global Data.vi" "gearDepthraw left"(w258) -> ()
    n188 = global write "Robot Global Data.vi" "encHopPos"(w290) -> ()
    n189 = global write "Robot Global Data.vi" "encHopSpeed"(w287) -> ()
    n190 = global write "Robot Global Data.vi" "gearSense raw"(w284) -> ()
    n191 = Negate(x=w270) -> (-x=w269:dbl)
    n192 = call-poly <vilib>:"NT Read Value.vi"("Name"="target_x") -> ("Numeric"=w267:dbl)  [unwired: 9 in, 1 out]
    n193 = call-poly <vilib>:"NT Read Value.vi"("Name"="auto") -> ("Numeric"=w264:dbl)  [unwired: 9 in, 1 out]
    n194 = global write "Robot Global Data.vi" "encXpos"(w271) -> ()
    n195 = Or(x=w256, y=w257) -> (x .or. y?=w255:bool)
    n196 = global write "Robot Global Data.vi" "encYpos"(w269) -> ()
    n197 = global write "Robot Global Data.vi" "center X"(w267) -> ()
    n198 = disable-structure shown="Disabled" {
      disable-tunnel: w264 -> [w294 _]
      frame Disabled {
        n199 = global write "Robot Global Data.vi" "auto"(w294) -> ()
      }
      frame Enabled {
      }
    }
    n200 = call-poly <vilib>:"NT Write Value.vi"("Boolean"=w255, "Name"="IR Distance") -> ()  [unwired: 9 in, 1 out]
    n201 = Greater?(x=w279, y="gearDepthresh right") -> (0:w280:bool)
    n202 = Greater?(x=w258, y="gearDepthresh left") -> (0:w259:bool)
    n203 = call-poly <vilib>:"NT Read Value.vi"("Name"="target_y") -> ("Numeric"=w268:dbl)  [unwired: 9 in, 1 out]
    n204 = Greater?(x=w284, y="gearSensthresh") -> (0:w282:bool)
    n205 = global write "Robot Global Data.vi" "gear Depth? right"(w280) -> ()
    n206 = global write "Robot Global Data.vi" "gear Depth? left"(w259) -> ()
    n207 = global write "Robot Global Data.vi" "center Y"(w268) -> ()
    n208 = global read "Robot Global Data.vi" "fieldcentric"() -> (w262:bool)
    n209 = global read "Robot Global Data.vi" "finished aim?"() -> (w265:bool)
    n210 = global write "Robot Global Data.vi" "have Gear?"(w282) -> ()
    n211 = call-poly <vilib>:"NT Write Value.vi"("Boolean"=w262, "Name"="drivemode") -> ()  [unwired: 9 in, 1 out]
    n212 = call-poly <vilib>:"NT Write Value.vi"("Boolean"=w265, "Name"="aimed") -> ()  [unwired: 9 in, 1 out]
    n213 = call-poly <vilib>:"NT Read Value.vi"("Name"="target_distance") -> ("Numeric"=w266:dbl)  [unwired: 9 in, 1 out]
    n214 = global write "Robot Global Data.vi" "target dist"(w266) -> ()
  }
  n215 = while {
    shift-right: [w298] -> _
    shift-left: 0 ("f") -> [w299]
    shift-left: 1 ("f") -> [w296]
    tunnel: w35 -> [w295]
    i -> [w297]
    stop <- FALSE stop-if-true
    # "gear stuff"
    n216 = Wait (ms)(milliseconds to wait=u32 20) -> ()  [unwired: 1 out]
    n217 = case shown="0, Default" w299 {
      selector: w299 -> [_ _ _ _ w370 _]
      tunnel: [w308 w324 w339 w350 w366 w378] -> w298
      tunnel: w297 -> [w302 w320 w335 w345 w365 w374]
      tunnel: w296 -> [_ _ _ _ _ w375]
      tunnel: w295 -> [w307 _ _ _ _ _]
      frame 1 {
        # "Reset encoder (for 3 loop cycles)"
        n218 = local read "timeSaved"() -> (w306:i32)
        n219 = local write "timeSaved 2"(w302) -> ()
        n220 = Subtract(x=w306, y=w302) -> (x-y=w303:i32)
        n221 = Absolute Value(x=w303) -> (abs(x)=w304:i32)
        n222 = Greater?(x=w304, y=3) -> (0:w314:bool)
        n223 = global read "Robot Global Data.vi" "Gear Eject"() -> (w311:bool)
        n224 = Select(t=3, s=w314, f=1) -> (s? t:f=w312:i32)
        n225 = call <vilib>:"WPI_EncoderReset.vi"("EncoderDevRef"=w307) -> ()  [unwired: 9 in, 2 out]
        n226 = Not(x=w311) -> (.not. x?=w310:bool)
        n227 = Select(t=0, s=w310, f=w312) -> (s? t:f=w308:i32)
      }
      frame 2 {
        n228 = local read "timeSaved 2"() -> (w321:i32)
        n229 = local write "timeSaved"(w320) -> ()
        n230 = Subtract(x=w321, y=w320) -> (x-y=w319:i32)
        n231 = Absolute Value(x=w319) -> (abs(x)=w318:i32)
        n232 = Greater?(x=w318, y="SHIMMYTIME1") -> (0:w316:bool)
        n233 = Select(t=5, s=w316, f=2) -> (s? t:f=w325:i32)
        n234 = global read "Robot Global Data.vi" "Gear Eject"() -> (w328:bool)
        n235 = local write "xshimmy"(TRUE ("xshimmy")) -> ()
        n236 = Not(x=w328) -> (.not. x?=w327:bool)
        n237 = Select(t=0, s=w327, f=w325) -> (s? t:f=w324:i32)
      }
      frame 5 {
        n238 = local write "timeSaved 2"(w335) -> ()
        n239 = local read "timeSaved"() -> (w336:i32)
        n240 = Subtract(x=w336, y=w335) -> (x-y=w334:i32)
        n241 = Absolute Value(x=w334) -> (abs(x)=w333:i32)
        n242 = Greater?(x=w333, y="SHIMMYTIME2") -> (0:w331:bool)
        n243 = Select(t=3, s=w331, f=5) -> (s? t:f=w340:i32)
        n244 = global read "Robot Global Data.vi" "Gear Eject"() -> (w343:bool)
        n245 = local write "shimmyspeed"(-0.2 ("shimmyspeed")) -> ()
        n246 = local write "xshimmy"(TRUE ("xshimmy")) -> ()
        n247 = Not(x=w343) -> (.not. x?=w342:bool)
        n248 = Select(t=0, s=w342, f=w340) -> (s? t:f=w339:i32)
      }
      frame 3 {
        n249 = local write "timeSaved"(w345) -> ()
        n250 = local read "timeSaved 2"() -> (w359:i32)
        n251 = local write "SEQ Retainer Open"(TRUE ("Gear Retainer")) -> ()
        n252 = Subtract(x=w359, y=w345) -> (x-y=w348:i32)
        n253 = Absolute Value(x=w348) -> (abs(x)=w347:i32)
        n254 = Greater?(x=w347, y="open retainer time") -> (0:w356:bool)
        n255 = Select(t=4, s=w356, f=3) -> (s? t:f=w351:i32)
        n256 = global read "Robot Global Data.vi" "Gear Eject"() -> (w354:bool)
        n257 = Not(x=w354) -> (.not. x?=w353:bool)
        n258 = local write "xshimmy"(FALSE ("xshimmy")) -> ()
        n259 = Select(t=0, s=w353, f=w351) -> (s? t:f=w350:i32)
      }
      frame 4 {
        n260 = local read "timeSaved"() -> (w364:i32)
        n261 = local write "Gear Shover"(TRUE ("Gear Shover")) -> ()
        n262 = Subtract(x=w364, y=w365) -> (x-y=w361:i32)
        n263 = Absolute Value(x=w361) -> (abs(x)=w362:i32)
        n264 = Greater?(x=w362, y="drop gear time") -> (0:w367:bool)
        n265 = Select(t=0, s=w367, f=w370) -> (s? t:f=w366:i32)
        n266 = local write "xshimmy"(FALSE ("xshimmy")) -> ()
      }
      frame 0, Default {
        n267 = local write "xshimmy"(FALSE ("xshimmy")) -> ()
        n268 = global read "Robot Global Data.vi" "Gear Eject"() -> (w371:bool)
        n269 = Not Equal To 0?(x=w375) -> (x != 0?=w376:bool)
        n270 = case shown="True" w376 {
          frame False {
          }
          frame True {
            n271 = local write "SEQ Retainer Open"(FALSE ("Gear Retainer")) -> ()
            n272 = local write "Gear Shover"(FALSE ("Gear Shover")) -> ()
          }
        }
        n273 = feedback #5() -> (w373:bool)  [unwired: 1 in]
        n274 = feedback-in #5(w371) -> ()
        n275 = Greater?(x=w371, y=w373) -> (0:w372:bool)
        n276 = Select(t=1, s=w372, f=0) -> (s? t:f=w378:i32)
        "timeSaved" <- w374
      }
    }
  }
  n277 = while {
    stop <- FALSE stop-if-true
    # "climber"
    n278 = Wait (ms)(milliseconds to wait=u32 20) -> ()  [unwired: 1 out]
  }
  n279 = while {
    tunnel: w18 -> [w387]
    stop <- FALSE stop-if-true
    # "gyro"
    n280 = Wait (ms)(milliseconds to wait=u32 5) -> ()  [unwired: 1 out]
    n281 = call "Z900_navX_Get_YPRHfH.vi"("navX Device"=w387) -> ("YRPHfH"=w391:T18)  [unwired: 7 in, 3 out]
    n282 = global read "Robot Global Data.vi" "resetgyro"() -> (w386:bool)
    n283 = Unbundle By Name(w391) -> ("Yaw"=w390:dbl, "Fused Heading"=w385:dbl)  [unwired: 3 out]
    n284 = global write "Robot Global Data.vi" "headingF"(w385) -> ()
    n285 = case shown="True" w386 {
      tunnel: w387 -> [_ w392]
      frame False {
      }
      frame True {
        n286 = call "Z900_navX_Set_ZeroYaw.vi"("navX Device"=w392) -> ()  [unwired: 9 in, 2 out]
      }
    }
    n287 = global write "Robot Global Data.vi" "heading"(w390) -> ()
  }
  n288 = while {
    tunnel: w25 -> [w404]
    stop <- FALSE stop-if-true
    # "hopper"
    n289 = Wait (ms)(milliseconds to wait=u32 20) -> ()  [unwired: 1 out]
    n290 = global read "Robot Global Data.vi" "Shot Distance"() -> (w395:bool)
    n291 = global read "Robot Global Data.vi" "hopper far"() -> (w393:dbl)
    n292 = global read "Robot Global Data.vi" "Spinup shooter"() -> (w397:bool)
    n293 = global read "Robot Global Data.vi" "Shoot!"() -> (w399:bool)
    n294 = Select(t=w393, s=w395, f="hopperSpeedClose") -> (s? t:f=w394:dbl)
    n295 = Absolute Value(x=w394) -> (abs(x)=w401:dbl)
    n296 = And(x=w399, y=w397) -> (x .and. y?=w398:bool)
    n297 = Negate(x=w401) -> (-x=w400:dbl)
    n298 = Select(t=w400, s=w398, f=0.0) -> (s? t:f=w403:dbl)
    n299 = call <vilib>:"WPI_MotorControlSetOutput.vi"("Output"=w403, "MotorControlDevRef"=w404) -> ()  [unwired: 7 in, 3 out]
  }
  n300 = while {
    tunnel: w44 -> [w436]
    stop <- FALSE stop-if-true
    n301 = global read "Robot Global Data.vi" "x"() -> (w434:dbl)
    n302 = global read "Robot Global Data.vi" "y"() -> (w409:dbl)
    n303 = global read "Robot Global Data.vi" "z"() -> (w441:dbl)
    n304 = Wait (ms)(milliseconds to wait=u32 20) -> ()  [unwired: 1 out]
    n305 = Square(x=w441) -> (x^2=w433:dbl)
    n306 = Sign(1:w441) -> (0:w432:dbl)
    n307 = global read "Robot Global Data.vi" "autoaim"() -> (w428:bool)
    n308 = Compound Arithmetic op=MULTIPLY(w433, w432, 0.8 ("value")) -> (w429:dbl)
    n309 = Select(t="shimmyspeed", s="xshimmy", f=w434) -> (s? t:f=w413:dbl)
    n310 = local read "aimBot"() -> (w427:dbl)
    n311 = global read "Robot Global Data.vi" "autoaim"() -> (w410:bool)
    n312 = global read "Robot Global Data.vi" "autoaim"() -> (w414:bool)
    n313 = Select(t=w427, s=w428, f=w429) -> (s? t:f=w426:dbl)
    n314 = global read "Robot Global Data.vi" "fieldcentric"() -> (w440:bool)
    n315 = Select(t=0.0, s=w410, f=w409) -> (s? t:f=w408:dbl)
    n316 = Select(t=0.0, s=w414, f=w413) -> (s? t:f=w411:dbl)
    n317 = global read "Robot Global Data.vi" "strafeStraight"() -> (w420:bool)
    n318 = Bundle("x"=w411, "y"=w408, "aimBot"=w426) -> (w430:cluster{"x":dbl, "y":dbl, "aimBot":dbl})  [unwired: 1 in]
    n319 = call "Soft Start.vi"("Joysticks"=w430, "Slew Rates"="Slews") -> ("X-axis drive"=w424:dbl, "Y-axis drive"=w422:dbl, "Z-axis drive"=w421:dbl)
    n320 = case shown="True" w440 {
      tunnel: [0.0 ("Gyro Angle") w456] -> w435
      frame False {
      }
      frame True {
        n321 = global read "Robot Global Data.vi" "heading"() -> (w456:dbl)
      }
    }
    n322 = case shown="True" w420 {
      tunnel: [w447 w448] -> w425
      tunnel: w424 -> [w447 w448]
      tunnel: [w446 0.0 ("Y-axis drive")] -> w423
      tunnel: w422 -> [w446 _]
      tunnel: [w445 w449] -> w417
      tunnel: w421 -> [w445 _]
      frame False {
        n323 = global read "Robot Global Data.vi" "heading"() -> (→"YavSaved":dbl)
      }
      frame True {
        n324 = global read "Robot Global Data.vi" "heading"() -> (w450:dbl)
        n325 = local read "YavSaved"() -> (w451:dbl)
        n326 = call-poly <vilib>:"PID.vi"("output range"=cluster{"output high":dbl, "output low":dbl} {"output high"=0.8, "output low"=-0.8}, "PID gains"="PID Strafe Straight", "process variable"=w450, "setpoint"=w451) -> ("output"=w449:dbl)  [unwired: 6 in, 1 out]
      }
    }
    n327 = call <vilib>:"WPI_Power Get PDP Voltage.vi"() -> ("voltage (V)"=w418:dbl)  [unwired: 14 in, 1 out]
    n328 = Divide(x=12.0, y=w418) -> (x/y=w415:dbl)
    n329 = Multiply(x=w417, y=w415) -> (x*y=w416:dbl)
    n330 = call-poly <vilib>:"WPI_RobotDriveHolonomicDrive.vi"("Rotation"=w416, "Gyro Angle"=w435, "Y"=w423, "X"=w425, "RobotDriveDevRef"=w436) -> ()  [unwired: 4 in, 3 out]
  }
  n331 = call <vilib>:"WPI_MotorControlRefNum Registry Get.vi"("refnum name"="intakeMotor") -> ("MotorControlDevRef"=w42:T10)  [unwired: 9 in, 1 out]
  n332 = call <vilib>:"WPI_SolenoidRefNum Registry Get.vi"("refnum name"="intakeArticulate") -> ("SolenoidDevRef"=w40:T2)  [unwired: 9 in, 1 out]
  n333 = while {
    tunnel: w20 -> [w462]
    tunnel: w19 -> [w460]
    stop <- FALSE stop-if-true
    n334 = global read "Robot Global Data.vi" "GEAR-SHOVER"() -> (w470:bool)
    n335 = global read "Robot Global Data.vi" "have Gear?"() -> (w468:bool)
    n336 = global read "Robot Global Data.vi" "GEAR-RETAINER"() -> (w471:bool)
    n337 = Wait (ms)(milliseconds to wait=u32 20) -> ()  [unwired: 1 out]
    n338 = Not(x=w468) -> (.not. x?=w466:bool)
    n339 = And(x=w466, y="ARM Retainer open") -> (x .and. y?=w467:bool)
    n340 = Or(x="Gear Shover", y=w470) -> (x .or. y?=w474:bool)
    n341 = Select(t=WPI_SolenoidValue."On" ("Value"), s=w474, f=WPI_SolenoidValue."Off" ("Value")) -> (s? t:f=w461:T19)
    n342 = Compound Arithmetic op=OR("SEQ Retainer Open", w471, w467) -> (w473:bool)
    n343 = feedback #6() -> (w464:T19)  [unwired: 1 in]
    n344 = feedback-in #6(w461) -> ()
    n345 = Select(t=WPI_SolenoidValue."On" ("Value"), s=w473, f=WPI_SolenoidValue."Off" ("Value")) -> (s? t:f=w457:T19)
    n346 = Not Equal?(x=w461, y=w464) -> (x != y?=w463:bool)
    n347 = case shown="True" w463 {
      tunnel: w461 -> [_ w484]
      tunnel: w462 -> [_ w483]
      frame False {
      }
      frame True {
        n348 = call-poly <vilib>:"WPI_SolenoidSet.vi"("Value"=w484, "SolenoidDevRef"=w483) -> ()  [unwired: 8 in, 2 out]
      }
    }
    n349 = feedback #7() -> (w459:T19)  [unwired: 1 in]
    n350 = feedback-in #7(w457) -> ()
    n351 = Not Equal?(x=w457, y=w459) -> (x != y?=w458:bool)
    n352 = case shown="True" w458 {
      tunnel: w460 -> [_ w482]
      tunnel: w457 -> [_ w481]
      frame False {
      }
      frame True {
        n353 = call-poly <vilib>:"WPI_SolenoidSet.vi"("Value"=w481, "SolenoidDevRef"=w482) -> ()  [unwired: 8 in, 2 out]
      }
    }
  }
  n354 = while {
    tunnel: w42 -> [w529]
    tunnel: w40 -> [w516]
    tunnel: w38 -> [w517]
    stop <- FALSE stop-if-true
    # "intake"
    n355 = global read "Robot Global Data.vi" "Arm Stow"() -> (w489:bool)
    n356 = global read "Robot Global Data.vi" "Intake"() -> (w487:bool)
    n357 = Wait (ms)(milliseconds to wait=u32 50) -> ()  [unwired: 1 out]
    n358 = Not(x=w489) -> (.not. x?=w486:bool)
    n359 = And(x=w487, y=w486) -> (x .and. y?=w485:bool)
    n360 = global read "Robot Global Data.vi" "Arm NUM"() -> (w495:i16)
    n361 = Select(t="intakeSpeed", s=w485, f=0.0) -> (s? t:f=w523:dbl)
    n362 = Equal?(x=i16 0 ("y"), y=w495) -> (x = y?=w509:bool)
    n363 = Equal?(x=w495, y=i16 2) -> (x = y?=w497:bool)
    n364 = Equal?(x=i16 1 ("y"), y=w495) -> (x = y?=w494:bool)
    n365 = local write "ARM Retainer open"(w494) -> ()
    n366 = call <vilib>:"WPI_MotorControlSetOutput.vi"("Output"=w523, "MotorControlDevRef"=w529) -> ()  [unwired: 7 in, 3 out]
    n367 = global read "Robot Global Data.vi" "Arm Stow"() -> (w498:bool)
    n368 = local read "panic"() -> (w490:bool)
    n369 = global read "Robot Global Data.vi" "Arm 1"() -> (w512:bool)
    n370 = global read "Robot Global Data.vi" "Arm 2"() -> (w513:bool)
    n371 = Compound Arithmetic op=OR(w494, w497, FALSE ("value")) -> (w502:bool)
    n372 = Compound Arithmetic op=OR(w509, w497, FALSE ("value")) -> (w508:bool)
    n373 = Not(x=w498) -> (.not. x?=w503:bool)
    n374 = Boolean To (0,1)(Boolean=w512) -> (0, 1=w514:i16)
    n375 = Boolean To (0,1)(Boolean=w513) -> (0, 1=w500:i16)
    n376 = And(x=w503, y=w502) -> (x .and. y?=w505:bool)
    n377 = And(x=w508, y=w503) -> (x .and. y?=w504:bool)
    n378 = Multiply(x=w500, y=i16 2) -> (x*y=w501:i16)
    n379 = Add(x=w514, y=w501) -> (x+y=w492:i16)
    n380 = Select(t=i16 1, s=w490, f=w492) -> (s? t:f=w493:i16)
    n381 = Select(t=WPI_SolenoidValue."On" ("Value"), s=w504, f=WPI_SolenoidValue."Off" ("Value")) -> (s? t:f=w524:T19)
    n382 = Select(t=WPI_SolenoidValue."On" ("Value"), s=w505, f=WPI_SolenoidValue."Off" ("Value")) -> (s? t:f=w515:T19)
    n383 = feedback-in #8(w524) -> ()
    n384 = feedback #8() -> (w526:T19)  [unwired: 1 in]
    n385 = feedback #9() -> (w519:T19)  [unwired: 1 in]
    n386 = feedback-in #9(w515) -> ()
    n387 = global write "Robot Global Data.vi" "Arm NUM"(w493) -> ()
    n388 = Not Equal?(x=w524, y=w526) -> (x != y?=w525:bool)
    n389 = Not Equal?(x=w515, y=w519) -> (x != y?=w518:bool)
    n390 = case shown="True" w525 {
      tunnel: w524 -> [_ w535]
      tunnel: w516 -> [_ w534]
      frame False {
      }
      frame True {
        n391 = call-poly <vilib>:"WPI_SolenoidSet.vi"("Value"=w535, "SolenoidDevRef"=w534) -> ()  [unwired: 8 in, 2 out]
      }
    }
    n392 = case shown="True" w518 {
      tunnel: w515 -> [_ w533]
      tunnel: w517 -> [_ w532]
      frame False {
      }
      frame True {
        n393 = call-poly <vilib>:"WPI_SolenoidSet.vi"("Value"=w533, "SolenoidDevRef"=w532) -> ()  [unwired: 8 in, 2 out]
      }
    }
  }
  n394 = call <vilib>:"WPI_MotorControlRefNum Registry Get.vi"("refnum name"="shooter3") -> ("MotorControlDevRef"=w3:T10)  [unwired: 9 in, 1 out]
  n395 = while {
    shift-right: [w570] -> _
    shift-left: 0 ("y") -> [w572]
    tunnel: w29 -> [w553]
    tunnel: w28 -> [w552]
    tunnel: w27 -> [w551]
    tunnel: w24 -> [w550]
    shift-right: [w546] -> _
    shift-left: _ -> [w545]
    tunnel: w3 -> [w537]
    i -> [w547]
    stop <- FALSE stop-if-true
    # "KILL IT IN DISABLED"
    n396 = global read "Robot Global Data.vi" "Spinup shooter"() -> (w571:bool)
    n397 = global read "Robot Global Data.vi" "Shot Distance"() -> (w554:bool)
    n398 = feedback #10() -> (w544:dbl[])  [unwired: 1 in]
    n399 = Delete From Array(array=w544, length=400) -> (deleted portion=w541:dbl[])  [unwired: 1 in, 1 out]
    n400 = Build Array (concatenate)(w541, w545) -> (w542:dbl[])
    n401 = feedback-in #10(w542) -> ()
    n402 = Wait (ms)(milliseconds to wait=u32 10) -> ()  [unwired: 1 out]
    n403 = global read "Robot Global Data.vi" "Trim Close Raw"() -> (w561:dbl)
    n404 = global read "Robot Global Data.vi" "Trim Far Raw"() -> (w563:dbl)
    n405 = case shown="3" w572 {
      selector: w572 -> [_ _ w626 w653 _]
      tunnel: w571 -> [w582 w599 w630 w652 _]
      tunnel: [w583 w595 w624 w651 w664] -> w570
      tunnel: [w577 w585 w601 w631 w660] -> w569
      tunnel: [w577 w585 w601 w631 w660] -> w568
      tunnel: w554 -> [_ w589 w627 w655 _]
      tunnel: w550 -> [w579 w588 w623 w650 _]
      tunnel: w547 -> [_ _ _ _ _]
      tunnel: [0.0 0.0 0.0 w638 0.0] -> w546
      tunnel: w542 -> [_ _ w604 w635 _]
      tunnel: [w577 w585 w601 w631 w660] -> w536
      frame 0, Default {
        w577 = 0.0
        # "1"
        # "Reset Ramp to 0"
        # "Shooter-off"
        n406 = call <vilib>:"WPI_CompressorStart.vi"("CompressorDevRef"=w579) -> ()  [unwired: 9 in, 2 out]
        n407 = local write "Ramp-Up"(0.0 ("Power")) -> ()
        n408 = Select(t=1 ("f"), s=w582, f=0 ("y")) -> (s? t:f=w583:i32)
      }
      frame 1 {
        # "Ramp motors based on Close"
        n409 = call <vilib>:"WPI_CompressorStop.vi"("CompressorDevRef"=w588) -> ()  [unwired: 9 in, 2 out]
        n410 = local read "feed forward close"() -> (w586:dbl)
        n411 = Add(x=0.005, y="Ramp-Up") -> (x+y=w585:dbl)
        n412 = local write "Ramp-Up"(w585) -> ()
        n413 = Select(t=1 ("f"), s=w599, f=4 ("y")) -> (s? t:f=w597:i32)
        n414 = Greater Or Equal?(x=w585, y=w586) -> (x >= y?=w596:bool)
        n415 = Select(t=3 ("y"), s=w589, f=2 ("y")) -> (s? t:f=w590:i32)
        n416 = Select(t=w590, s=w596, f=w597) -> (s? t:f=w595:i32)
        n417 = global write "Robot Global Data.vi" "ramp down"(w585) -> ()
      }
      frame 2 {
        # "PID Close"
        n418 = call <vilib>:"WPI_CompressorStop.vi"("CompressorDevRef"=w623) -> ()  [unwired: 9 in, 2 out]
        n419 = Select(t=3, s=w627, f=w626) -> (s? t:f=w625:i32)
        n420 = global read "Robot Global Data.vi" "Trim Far"() -> (w617:dbl)
        n421 = global read "Robot Global Data.vi" "encShootSpeed"() -> (w611:dbl)
        n422 = Select(t=w625, s=w630, f=4) -> (s? t:f=w624:i32)
        n423 = Multiply(x="shooter target speed close", y=w617) -> (x*y=w610:dbl)
        n424 = global read "Robot Global Data.vi" "Trim Far"() -> (w606:dbl)
        n425 = call "CustomPID_v2.1.vi"("Kp"="Kp 2", "Process Variable"=w611, "Goal"=w610, "Ki"="Ki 2", "Kd"="Kd 2", "Max Ouput"=0.5, "Min Output"=-0.4) -> ("Command"=w608:dbl)  [unwired: 6 in, 2 out]
        n426 = Multiply(x="feed forward close", y=w606) -> (x*y=w605:dbl)
        n427 = call <vilib>:"WPI_Power Get PDP Voltage.vi"() -> ("voltage (V)"=w620:dbl)  [unwired: 14 in, 1 out]
        n428 = Divide(x=12.0, y=w620) -> (x/y=w619:dbl)
        n429 = Multiply(x=w605, y=w619) -> (x*y=w618:dbl)
        n430 = Add(x=w608, y=w618) -> (x+y=w601:dbl)
        n431 = global write "Robot Global Data.vi" "ramp down"(w601) -> ()
        n432 = call <vilib>:"Std Deviation and Variance.vi"("X"=w604) -> ("mean"=w602:dbl, "standard deviation"=w603:dbl)  [unwired: 1 in, 1 out]
        n433 = local write "Waveform Graph"(w604) -> ()
        n434 = local write "std dev"(w603) -> ()
        n435 = local write "mean"(w602) -> ()
      }
      frame 3 {
        # "PID Far"
        n436 = call <vilib>:"WPI_CompressorStop.vi"("CompressorDevRef"=w650) -> ()  [unwired: 9 in, 2 out]
        n437 = global read "Robot Global Data.vi" "encShootSpeed"() -> (w638:dbl)
        n438 = Select(t=w653, s=w655, f=2 ("t")) -> (s? t:f=w656:i32)
        n439 = global read "Robot Global Data.vi" "Trim Far"() -> (w658:dbl)
        n440 = global read "Robot Global Data.vi" "feed forward far"() -> (w632:dbl)
        n441 = Select(t=w656, s=w652, f=4) -> (s? t:f=w651:i32)
        n442 = Multiply(x="shooter target speed far", y=w658) -> (x*y=w644:dbl)
        n443 = global read "Robot Global Data.vi" "Trim Far"() -> (w637:dbl)
        n444 = call <vilib>:"WPI_Power Get PDP Voltage.vi"() -> ("voltage (V)"=w648:dbl)  [unwired: 14 in, 1 out]
        n445 = call "CustomPID_v2.1.vi"("Kp"="Kp", "Process Variable"=w638, "Goal"=w644, "Ki"="Ki", "Kd"="Kd", "Max Ouput"=0.5, "Min Output"=-0.4) -> ("Command"=w645:dbl)  [unwired: 6 in, 2 out]
        n446 = Multiply(x=w632, y=w637) -> (x*y=w636:dbl)
        n447 = Divide(x=12.0, y=w648) -> (x/y=w647:dbl)
        n448 = Multiply(x=w636, y=w647) -> (x*y=w646:dbl)
        n449 = Add(x=w645, y=w646) -> (x+y=w631:dbl)
        n450 = global write "Robot Global Data.vi" "ramp down"(w631) -> ()
        n451 = call <vilib>:"Std Deviation and Variance.vi"("X"=w635) -> ("mean"=→"mean":dbl, "standard deviation"=→"std dev":dbl)  [unwired: 1 in, 1 out]
        "Waveform Graph" <- w635
      }
      frame 4 {
        # "Ramp motors based on Close"
        n452 = global read "Robot Global Data.vi" "ramp down"() -> (w661:dbl)
        n453 = Add(x=-0.005, y=w661) -> (x+y=w660:dbl)
        n454 = global write "Robot Global Data.vi" "ramp down"(w660) -> ()
        n455 = Less Or Equal To 0?(x=w660) -> (x <= 0?=w663:bool)
        n456 = Select(t=0 ("f"), s=w663, f=4 ("y")) -> (s? t:f=w664:i32)
      }
    }
    n457 = Select(t=WPI_SolenoidValue."On" ("Value"), s=w554, f=WPI_SolenoidValue."Off" ("Value")) -> (s? t:f=w559:T19)
    n458 = feedback #11() -> (w557:T19)  [unwired: 1 in]
    n459 = feedback-in #11(w559) -> ()
    n460 = Multiply(x=w561, y=0.02 ("value")) -> (x*y=w564:dbl)
    n461 = Multiply(x=w563, y=-0.02 ("value")) -> (x*y=w567:dbl)
    n462 = Not Equal?(x=w559, y=w557) -> (x != y?=w558:bool)
    n463 = Add(x=w564, y=1.0) -> (x+y=w548:dbl)
    "trim close" <- w548
    n464 = Add(x=w567, y=1.0) -> (x+y=w549:dbl)
    "trim far" <- w549
    n465 = case shown="True" w558 {
      tunnel: w559 -> [_ w576]
      tunnel: w553 -> [_ w575]
      frame False {
      }
      frame True {
        n466 = call-poly <vilib>:"WPI_SolenoidSet.vi"("Value"=w576, "SolenoidDevRef"=w575) -> ()  [unwired: 8 in, 2 out]
      }
    }
    n467 = global write "Robot Global Data.vi" "Trim Close"(w548) -> ()
    n468 = global write "Robot Global Data.vi" "Trim Far"(w549) -> ()
    n469 = call <vilib>:"WPI_Power Get PCM Voltage.vi"() -> ("Input Voltage"=→"Input Voltage":dbl)  [unwired: 13 in, 2 out]
    n470 = call <vilib>:"WPI_Power Get PDP Voltage.vi"("Power Distribution Panel (0)"=u8 0) -> ("voltage (V)"=→"voltage (V)":dbl)  [unwired: 13 in, 1 out]
    n471 = call <vilib>:"WPI_MotorControlSetOutput.vi"("Output"=w569, "MotorControlDevRef"=w552) -> ()  [unwired: 7 in, 3 out]
    n472 = call <vilib>:"WPI_MotorControlSetOutput.vi"("Output"=w568, "MotorControlDevRef"=w551) -> ()  [unwired: 7 in, 3 out]
    n473 = call <vilib>:"WPI_MotorControlSetOutput.vi"("Output"=w536, "MotorControlDevRef"=w537) -> ()  [unwired: 7 in, 3 out]
  }
